vi "save.vi"(8 "error in (no error)":errorcluster, 9 "base name":string, 10 "folder path":path, 11 "DataCollectionDL110128Streaming in":refnum<class "DataCollectionDL110128Streaming.lvclass">) -> (0 "error out":errorcluster, 3 "DataCollectionDL110128Streaming out":refnum<class "DataCollectionDL110128Streaming.lvclass">)   [LabVIEW 2010, in "DataCollectionDL110128Streaming.lvclass"]
uses:
  DataCollectionDL110128Streaming.lvclass
  DataCollectionDL091104Scaffold/DataCollectionDL091104Scaffold/DataCollectionDL091104Scaffold.lvclass
  DataCollectionDL110128Streaming.lvclass/DataCollectionDL110128Streaming.ctl
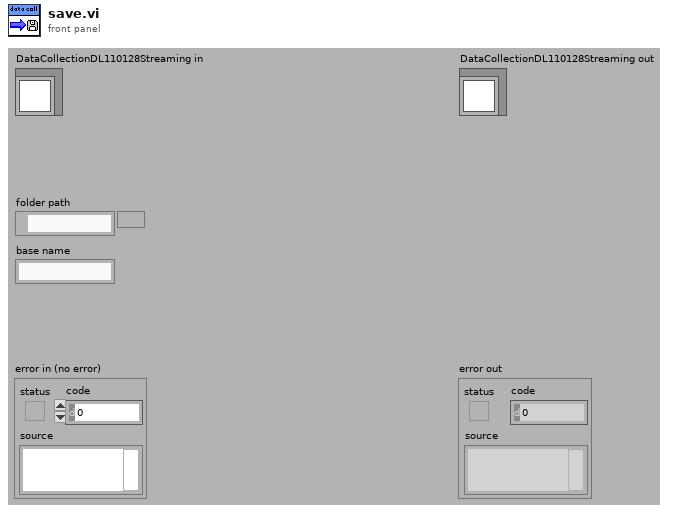
[diagram p1: front panel]
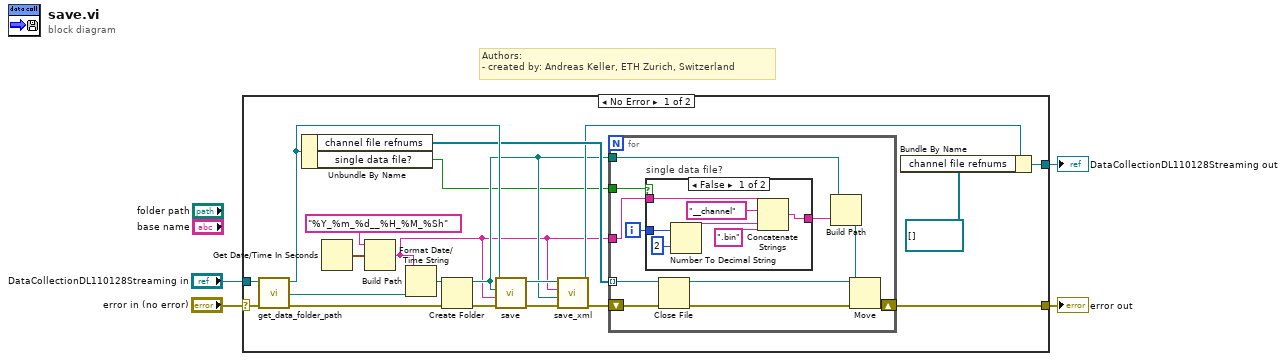
[diagram p0: block diagram]
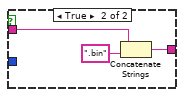
[diagram p2: hidden frame]
diagram:
  # "Authors: \n- created by: Andreas Keller, ETH Zurich, Switzerland"
  n1 = case shown="No Error" "error in (no error)" {
    selector: "error in (no error)" -> [w24 w47]
    tunnel: [w13 w47] -> w4
    tunnel: [w17 w46] -> w3
    tunnel: "DataCollectionDL110128Streaming in" -> [w23 w46]
    frame No Error {
      n2 = call-dynamic "get_data_folder_path.vi"("error in (no error)"=w24, "GenericComponent in"=w23) -> ("error out"=w18:errorcluster, "data folder path"=w20:path, "GenericComponent out"=w14:refnum<class "DataCollectionDL110128Streaming.lvclass">)  [unwired: 7 out]
      n3 = Unbundle By Name(w14) -> ("channel file refnums"=w10:refnum<file>[], "single data file?"=w5:bool)
      n4 = Get Date/Time In Seconds() -> (seconds since 1Jan1904=w21:timestamp)
      n5 = Format Date/Time String(time format string (%c)="%Y_%m_%d__%H_%M_%Sh", seconds (now)=w21) -> (date/time string=w6:string)  [unwired: 1 out]
      n6 = Build Path(base path=w20, name or relative path=w6) -> (appended path=w19:path)
      n7 = Create Folder(path (use dialog)=w19, error in=w18) -> (created path=w7:path, error out=w15:errorcluster)  [unwired: 1 in, 1 out]
      n8 = call-parent "save.vi"("error in (no error)"=w15, "base name"=w6, "folder path"=w7, "DL090215DataCollection in"=w14) -> ("error out"=w12:errorcluster, "DL090215DataCollection out"=w9:refnum<class "DataCollectionDL110128Streaming.lvclass">)  [unwired: 6 in]
      n9 = call-dynamic "save_xml.vi"("error in (no error)"=w12, "appended path"=w7, "string"=w6, "DataCollectionDL110128Streaming in"=w9) -> ("error out"=w11:errorcluster, "DataCollectionDL110128Streaming out"=w8:refnum<class "DataCollectionDL110128Streaming.lvclass">)  [unwired: 6 in]
      n10 = for {
        tunnel: w10 -> [w35] mode=indexing
        shift-right: [w28] -> w13
        shift-left: w11 -> [w29]
        tunnel: w7 -> [w27]
        tunnel: w6 -> [w26]
        tunnel: w5 -> [w25]
        i -> [w32]
        n11 = case "single data file?" shown="False" w25 {
          tunnel: w32 -> [w39 _]
          tunnel: [w38 w45] -> w31
          tunnel: w26 -> [w36 w44]
          frame False {
            n12 = Number To Decimal String(number=w39, width (-)=i16 2) -> (decimal integer string=w41:string)
            n13 = Concatenate Strings(w36, "__channel" ("string"), w41, ".bin" ("string")) -> (w38:string)
          }
          frame True {
            n14 = Concatenate Strings(w44, ".bin" ("string")) -> (w45:string)
          }
        }
        n15 = Close File(refnum=w35, error in=w29) -> (path=w33:path, error out=w34:errorcluster)
        n16 = Build Path(base path=w27, name or relative path=w31) -> (appended path=w30:path)
        n17 = Move(source path=w33, error in=w34, 10:w30) -> (error out=w28:errorcluster)  [unwired: 2 in, 2 out]
      }
      n18 = Bundle By Name(cluster=w8, "channel file refnums"=refnum<file>[] []) -> (w17:refnum<class "DataCollectionDL110128Streaming.lvclass">)
    }
    frame Error {
    }
  }
  "error out" <- w4
  "DataCollectionDL110128Streaming out" <- w3
